vi "pmu_CRC-CCIT.vi"(7 "byte array":u8[](array[numeric]) format="%x") -> (4 "CRCbytes":u8[](array[numeric]), 8 "CRC-CCIT":u16 format="%.0x")   [LabVIEW 2011, in "NI_EP_PMU.lvlib"]
uses:
  <vilib>/addons/Electrical Power/PMU/NI_EP_PMU.lvlib
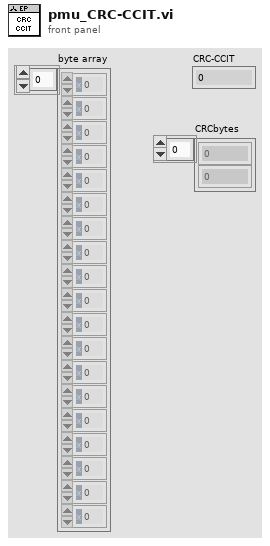
[diagram p1: front panel]
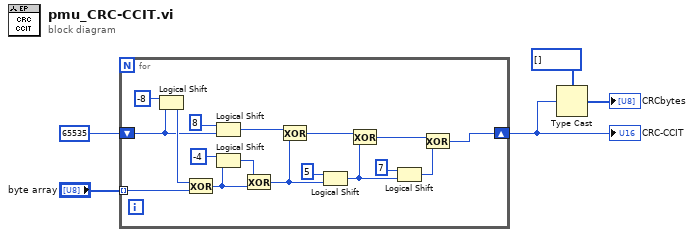
[diagram p0: block diagram]
diagram:
  n1 = for {
    tunnel: "byte array" -> [w20] mode=indexing
    shift-right: [w6] -> w3
    shift-left: u16 65535 -> [w19]
    n2 = Logical Shift(y=i8 -8, x=w19) -> (x << y=w21:u16)
    n3 = Exclusive Or(1:w20, 2:w21) -> (0:w16:u16)
    n4 = Logical Shift(y=i8 8, x=w19) -> (x << y=w14:u16)
    n5 = Logical Shift(y=i8 -4, x=w16) -> (x << y=w15:u16)
    n6 = Exclusive Or(1:w16, 2:w15) -> (0:w13:u16)
    n7 = Exclusive Or(1:w13, 2:w14) -> (0:w11:u16)
    n8 = Logical Shift(y=i8 5, x=w13) -> (x << y=w9:u16)
    n9 = Exclusive Or(1:w9, 2:w11) -> (0:w8:u16)
    n10 = Logical Shift(y=i8 7, x=w9) -> (x << y=w7:u16)
    n11 = Exclusive Or(1:w7, 2:w8) -> (0:w6:u16)
  }
  "CRC-CCIT" <- w3
  n12 = Type Cast(type=u8[] [], x=w3) -> (*(type *) &x=→"CRCbytes":u8[])
